vi "Create Folder if Not Present.vi"(8 "error in (no error)":errorcluster, 11 "Path":path) -> (0 "error out":errorcluster, 3 "Path out":path)   [LabVIEW 2016, in "SLL File IO.lvlib"]
doc: "Creates the folders for the given path, if not present."
uses:
  SLL File IO.lvlib
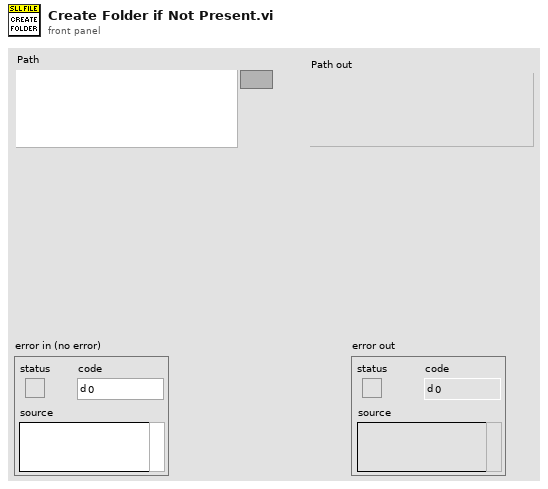
[diagram p1: front panel]
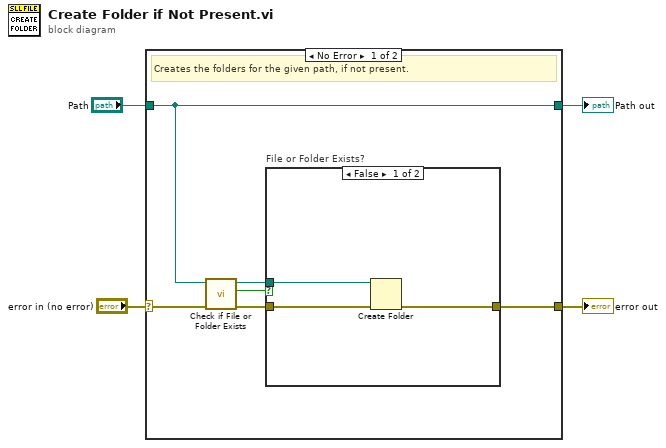
[diagram p0: block diagram]
diagram:
  n1 = case shown="No Error" "error in (no error)" {
    selector: "error in (no error)" -> [w10 w16]
    tunnel: [w9 w16] -> w3
    tunnel: "Path" -> [w5 w15]
    tunnel: [w5 w15] -> w1
    frame No Error {
      # "Creates the folders for the given path, if not present."
      n2 = call <vilib>:"Check if File or Folder Exists.vi"("error in (no error)"=w10, "path"=w5) -> ("error out"=w8:errorcluster, "file or folder exists?"=w7:bool, "dup path"=w6:path)  [unwired: 7 in]
      n3 = case "File or Folder Exists?" shown="False" w7 {
        tunnel: [w12 w14] -> w9
        tunnel: w8 -> [w13 w14]
        tunnel: w6 -> [w11 _]
        frame False {
          n4 = Create Folder(path (use dialog)=w11, error in=w13) -> (error out=w12:errorcluster)  [unwired: 1 in, 2 out]
        }
        frame True {
        }
      }
    }
    frame Error {
    }
  }
  "error out" <- w3
  "Path out" <- w1
